vi "Generate Signal.vi"(11 "User Specified":T1={"Hardware Configuration"={"Signal Channel"="PXI1Slot7/ao0", "Response Channel"="PXI1Slot7/ai0", "Trigger Channel"="/PXI1Slot7/PFI0", "Number of acquisitions"=0.0}, "Analysis Configuration"={"Statistics"=TRUE}, "Signal Type"=enum."Single Chirp", "New Data Behavior"=enum."Replace", "Signal Configuration"={"Chirp Amplitude"=0.1, "I/O Limit"=10.0, "Sample Rate"=1000000.0, "Chirp Duration (s)"=10000000.0, "Upper Frequency"=0.0, "Lower Frequency"=0.0, "Windowing"=enum."None"}}) -> (0 "Number of samples":dbl format="%0.2f", 1 "Y min":dbl format="%0.2f", 2 "Y max":dbl format="%0.2f", 3 "Final Waveform":waveform(dbl)(graph))   [LabVIEW 2017]
uses:
  controls/User Specified Data.ctl
  controls/HW Configuration.ctl
  controls/Analysis Configuration.ctl
  controls/New Data Behavior.ctl
  controls/Signal Configuration.ctl
  <vilib>/Waveform/WDTOps.llb/WDT Append Waveforms DBL.vi
  <vilib>/Waveform/WDTOps.llb/WDT Number of Waveform Samples DBL.vi
panel:
  out "Initial waveform":waveform(dbl)
  out "Shift register waveform":waveform(dbl)(graph)
  out "Number of rows":i32
  out "Voltage Offset":dbl
  out "Single Chirp w/ offset":waveform(dbl)(graph)
  out "Samples per chirp":dbl
  out "Single Chirp (Excel)":waveform(dbl)(graph)
  out "error out":errorcluster
  in  "error in":errorcluster
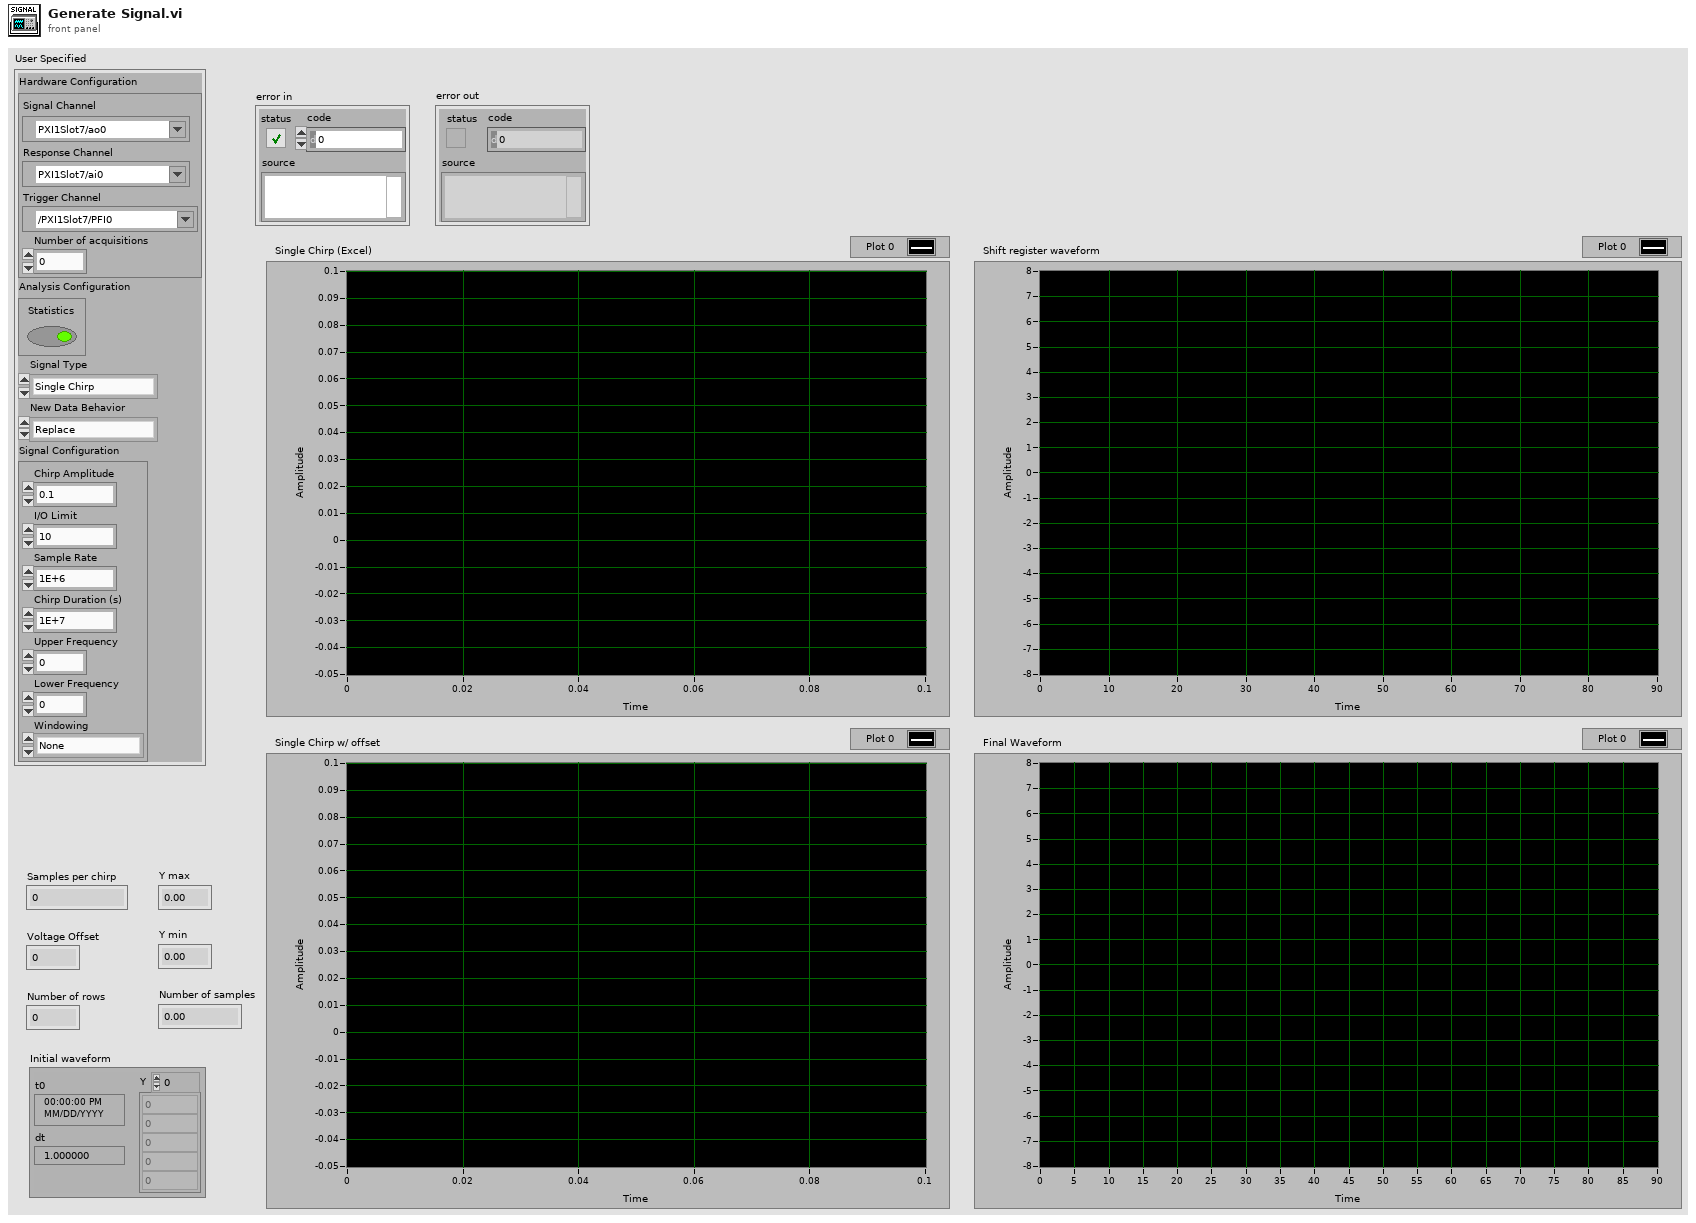
[diagram p1: front panel]
types:
  T1 = typedef "User Specified Data.ctl" = cluster{"Hardware Configuration":T2, "Analysis Configuration":T3, "Signal Type":enum16{"Single Chirp", "From Excel"}, "New Data Behavior":T4, "Signal Configuration":T5}
  T2 = typedef "HW Configuration.ctl" = cluster{"Signal Channel":tag, "Response Channel":tag, "Trigger Channel":tag, "Number of acquisitions":dbl}
  T3 = typedef "Analysis Configuration.ctl" = cluster{"Statistics":bool}
  T4 = typedef "New Data Behavior.ctl" = enum16{"Replace", "Overlay", "Append"}
  T5 = typedef "Signal Configuration.ctl" = cluster{"Chirp Amplitude":dbl, "I/O Limit":dbl, "Sample Rate":dbl, "Chirp Duration (s)":dbl, "Upper Frequency":dbl, "Lower Frequency":dbl, "Windowing":enum16{"None", "Exponential", "Flat top", "Hamming", "Hanning", "Kaiser-Bessel", "Rectangular"}}
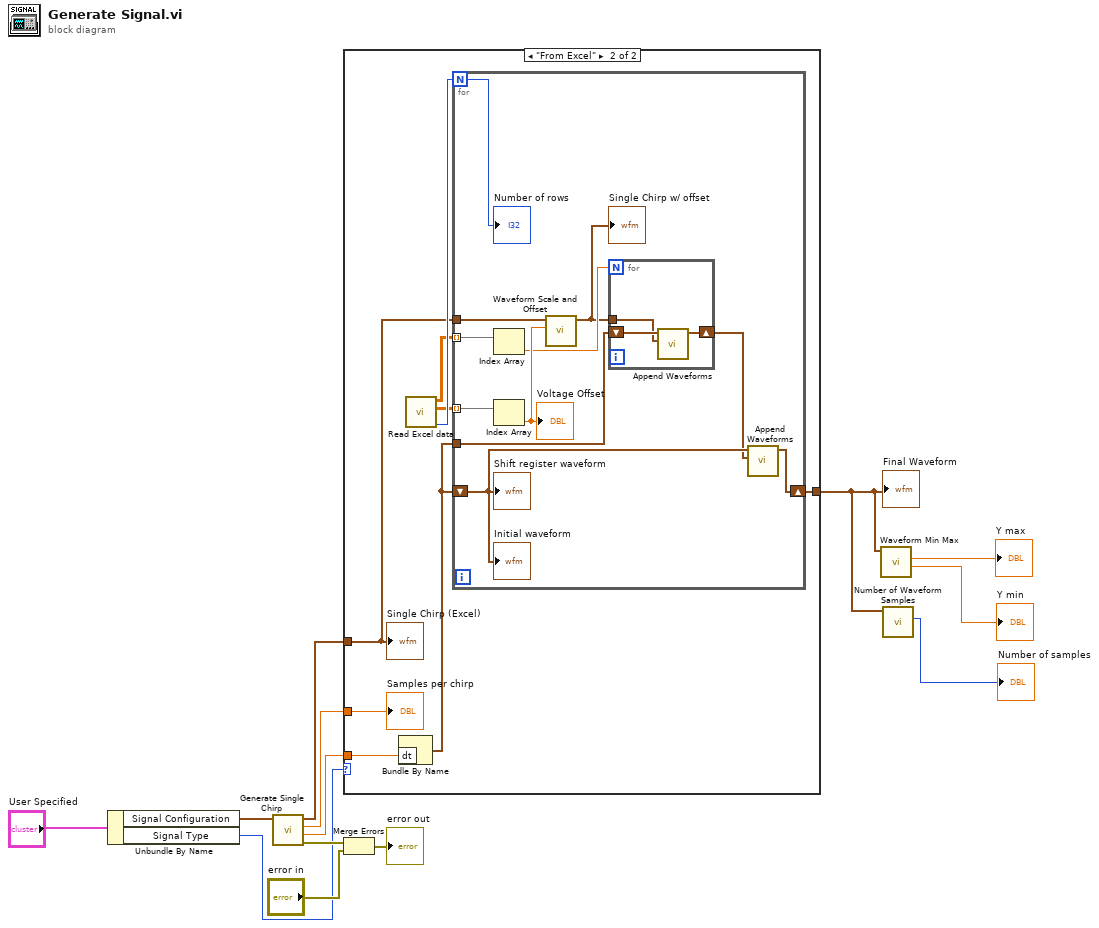
[diagram p0: block diagram]
diagram:
  n1 = Unbundle By Name("User Specified") -> ("Signal Configuration"=w10:T5, "Signal Type"=w9:enum16{"Single Chirp", "From Excel"})
  n2 = call "Generate Single Chirp.vi"("Signal Configuration"=w10) -> ("error out"=w11:errorcluster, "dt"=w1:dbl, "Number of samples"=w8:dbl, "Chirp"=w7:waveform(dbl))  [unwired: 7 in]
  n3 = case shown="\"From Excel\"" w9 {
    tunnel: w7 -> [w14 w18]
    tunnel: w8 -> [_ w22]
    tunnel: w1 -> [_ w17]
    tunnel: [w14 w15] -> w3
    frame "Single Chirp", Default {
    }
    frame "From Excel" {
      n4 = Bundle By Name("dt"=w17) -> (w16:waveform(dbl))  [unwired: 1 in]
      n5 = call "Read Excel data.vi"() -> ("Number of rows"=w21:i32, "Voltage Offsets"=w20:dbl[][], "Chirp Durations"=w19:dbl[][])  [unwired: 8 in, 1 out]
      n6 = for {
        N: w21 -> [w30]
        tunnel: w18 -> [w33]
        tunnel: w20 -> [w32] mode=indexing
        tunnel: w19 -> [w29] mode=indexing
        shift-right: [w28] -> w15
        shift-left: w16 -> [w27]
        tunnel: w16 -> [w24]
        n7 = Index Array(array=w29) -> (element=w26:dbl)  [unwired: 1 in]
        n8 = Index Array(array=w32) -> (element=w31:dbl)  [unwired: 1 in]
        "Voltage Offset" <- w31
        n9 = call <vilib>:"Waveform Scale and Offset.vi"("offset"=w31, "waveform in"=w33) -> ("waveform out"=w25:waveform(dbl))  [unwired: 8 in, 1 out]
        "Single Chirp w/ offset" <- w25
        n10 = for {
          N: w26 -> [_]
          tunnel: w25 -> [w35]
          shift-right: [w34] -> w23
          shift-left: w24 -> [w36]
          n11 = call-poly <vilib>:"Append Waveforms.vi"("waveform B"=w35, "waveform A"=w36) -> ("waveform out"=w34:waveform(dbl))  [unwired: 8 in, 1 out]
        }
        n12 = call-poly <vilib>:"Append Waveforms.vi"("waveform B"=w23, "waveform A"=w27) -> ("waveform out"=w28:waveform(dbl))  [unwired: 8 in, 1 out]
        "Number of rows" <- w30
        "Shift register waveform" <- w27
        "Initial waveform" <- w27
      }
      "Single Chirp (Excel)" <- w18
      "Samples per chirp" <- w22
    }
  }
  "Final Waveform" <- w3
  n13 = Merge Errors(w11, "error in") -> (→"error out":errorcluster)
  n14 = call <vilib>:"Waveform Min Max.vi"("waveform in"=w3) -> ("Y min"=→"Y min":dbl, "Y max"=→"Y max":dbl)  [unwired: 5 in, 4 out]
  n15 = call-poly <vilib>:"Number of Waveform Samples.vi"("waveform in"=w3) -> ("number of samples"=→"Number of samples":i32)  [unwired: 8 in, 2 out]
